vi "d1000 out bit.vi"(10 "BitData":i16, 11 "BitNo":i16) -> (3 "function return":u32)   [LabVIEW 2019, in "Dmc1000.lvlib"]
doc: "DMC1000_API DWORD WINAPI d1000_out_bit(short BitNo,short BitData);"
uses:
  Dmc1000.lvlib
  Dmc1000.dll
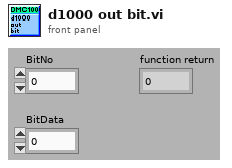
[diagram p1: front panel]
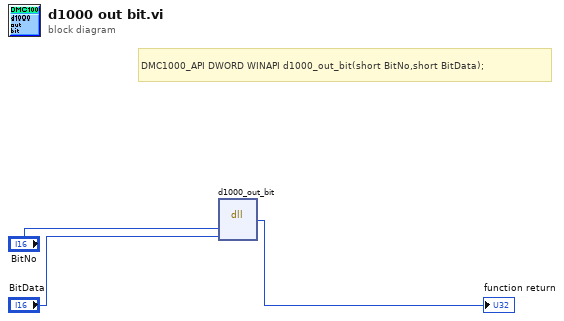
[diagram p0: block diagram]
diagram:
  # "DMC1000_API DWORD WINAPI d1000_out_bit(short BitNo,short BitData);"
  n1 = dll-call lib="C:/Users/VIC/Desktop/Standar Program/System/LLB/DMC1000B/Dmc1000.*" fn="d1000_out_bit"("BitNo"="BitNo", "BitData"="BitData") -> (→"function return":u32)  [unwired: 5 in, 2 out]
